vi "scanallvalues_clip.vi"(0 "VISA resource name out":refnum<visa-resource-name>, 1 "nm ch":i32[](array[numeric]), 2 "Voltages values":dbl[](array[numeric]), 3 "Init clip value":i32[](array[numeric]), 4 "base path":path, 5 "error in":errorcluster, 6 "Integration Board IP":string, 7 "L1 Address":i32, 8 "Save test data":bool=TRUE, 9 "Ch burst":i32, 11 "Init att value":i32[](array[numeric])) -> (14 "50%":dbl[][][][](array[numeric]), 15 "L1 min values":i32[](array[numeric])=[180, 378, 779, 1613, 2478, 4286, 5228, 6743], 19 "error out":errorcluster)   [LabVIEW 2009]
uses:
  <instrlib>/Agilent 81150/Agilent 81150.lvlib
  <vilib>/Analysis/NI_AALPro.lvlib
panel:
  out "State":i16
  out "Data out":string="ACK\r\n"
  out "XY Graph":cluster{"Y":dbl[], "Y":dbl[]}[](graph)
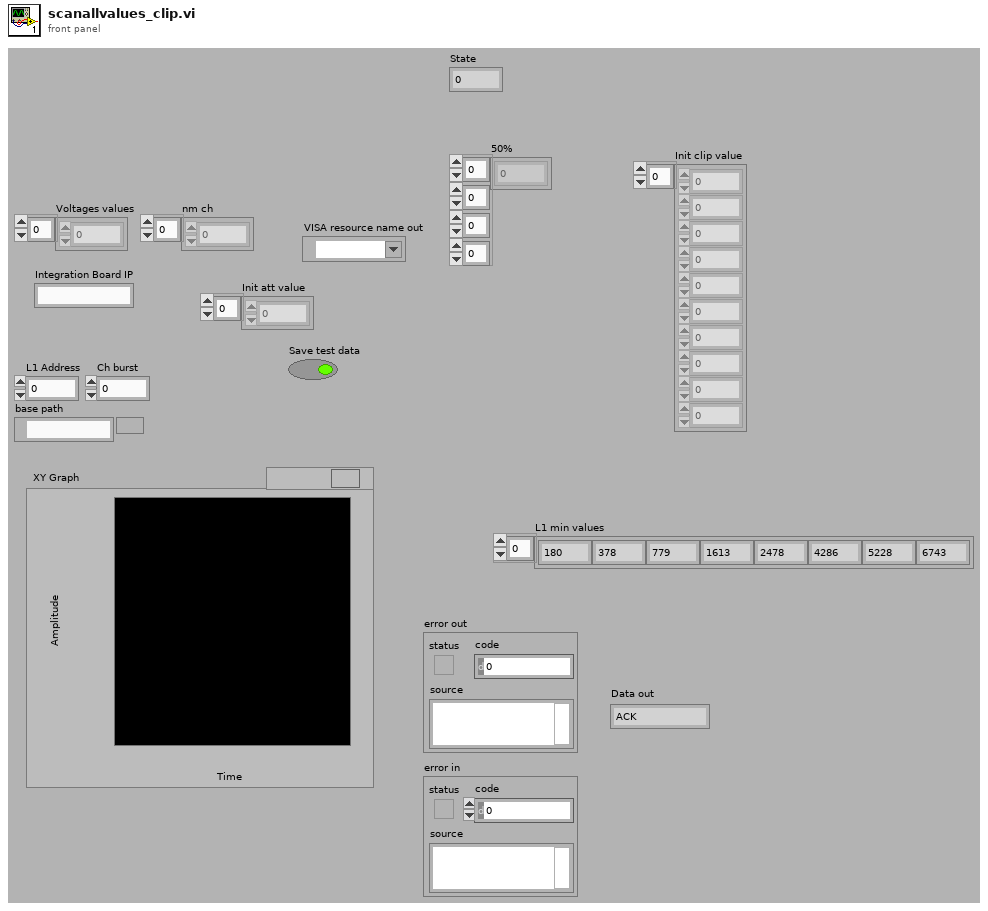
[diagram p1: front panel]
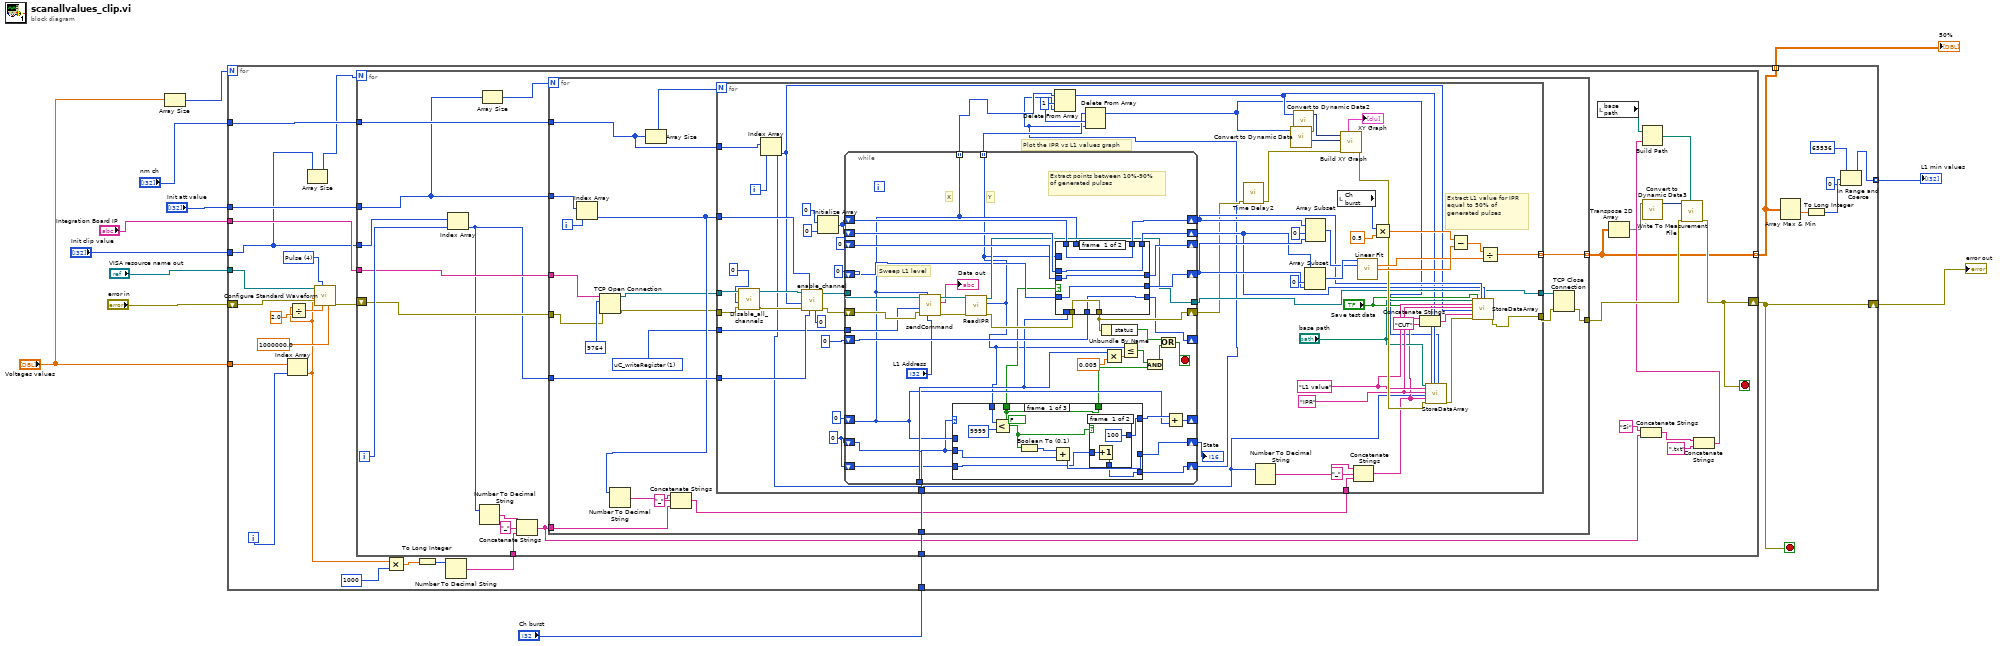
[diagram p0: block diagram]
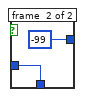
[diagram p2: hidden frame]
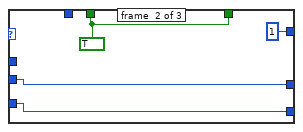
[diagram p3: hidden frame]
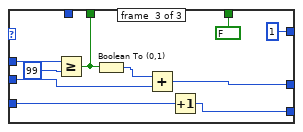
[diagram p4: hidden frame]
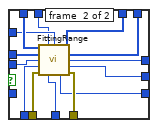
[diagram p5: hidden frame]
diagram:
  n1 = Array Size(array="Voltages values") -> (size(s)=w5:i32)
  n2 = for {
    N: w5 -> [_]
    shift-right: [w26] -> w11
    shift-left: "error in" -> [w25]
    tunnel: [w32] -> w10 mode=indexing
    tunnel: [w28] -> w1 mode=indexing
    tunnel: "Integration Board IP" -> [w27]
    tunnel: "VISA resource name out" -> [w29]
    tunnel: "Voltages values" -> [w19]
    tunnel: "Init clip value" -> [w13]
    tunnel: "Ch burst" -> [w18]
    tunnel: "nm ch" -> [w17]
    tunnel: "Init att value" -> [w15]
    i -> [w34]
    stop <- w26 stop-if-true
    w38 = u16 4 items=["Sine", "Square", "Ramp Up", "Ramp Down", "Pulse", "Noise", "DC"] ("Waveform (0: Sine)")
    n3 = Index Array(array=w19, index=w34) -> (element=w22:dbl)
    n4 = Divide(x=w22, y=2.0) -> (x/y=w36:dbl)
    n5 = Array Size(array=w13) -> (size(s)=w16:i32)
    n6 = call <instrlib>:"Configure Standard Waveform.vi"("Frequency (1000.0 Hz)"=1000000.0, "DC Offset (0.0 Volts)"=w36, "Waveform (0: Sine)"=w38, "error in (no error)"=w25, "Amplitude (1.0 Vpp)"=w22, "VISA resource name"=w29) -> ("error out"=w24:errorcluster)  [unwired: 4 in, 1 out]
    n7 = Multiply(x=w22, y=1000) -> (x*y=w21:dbl)
    n8 = To Long Integer(number=w21) -> (32bit integer=w20:i32)
    n9 = Number To Decimal String(number=w20) -> (decimal integer string=w14:string)  [unwired: 1 in]
    n10 = for {
      N: w16 -> [_]
      tunnel: [w41] -> w28 mode=indexing
      shift-right: [w55] -> w26
      shift-left: w24 -> [w60]
      tunnel: w27 -> [w61]
      tunnel: w13 -> [w43]
      tunnel: w18 -> [w62]
      tunnel: w17 -> [w59]
      tunnel: w15 -> [w42]
      tunnel: w14 -> [w52]
      i -> [w63]
      stop <- w55 stop-if-true
      n11 = Index Array(array=w43, index=w63) -> (element=w54:i32)
      n12 = Number To Decimal String(number=w54) -> (decimal integer string=w51:string)  [unwired: 1 in]
      n13 = Array Size(array=w42) -> (size(s)=w58:i32)
      n14 = Concatenate Strings(w51, "_" ("string"), w52) -> (w44:string)
      n15 = for {
        N: w58 -> [_]
        tunnel: [w84] -> w41 mode=indexing
        tunnel: w62 -> [w83]
        tunnel: [w68] -> w56
        tunnel: w61 -> [w81]
        tunnel: w60 -> [w80]
        tunnel: w59 -> [w76]
        tunnel: w42 -> [w79]
        tunnel: w54 -> [w75]
        tunnel: w44 -> [w73]
        i -> [w78]
        w66 = u16 1 items=["sendCommand"=9, "FPGA_writeRegister"=3, "FPGA_readRegister"=2, "uC_writeRegister"=1, "uC_readRegister"=0] ("Action")
        n16 = Index Array(array=w79, index=w78) -> (element=w74:i32)
        n17 = TCP Open Connection(address=w81, remote port or service name=u16 9764, error in (no error)=w80) -> (connection ID=w64:refnum<k5>, error out=w65:errorcluster)  [unwired: 2 in]
        n18 = Number To Decimal String(number=w74) -> (decimal integer string=w72:string)  [unwired: 1 in]
        n19 = Array Size(array=w76) -> (size(s)=w77:i32)
        n20 = Concatenate Strings(w72, "_" ("string"), w73) -> (w70:string)
        n21 = for {
          N: w77 -> [_]
          tunnel: [w97] -> w84 mode=indexing
          tunnel: w83 -> [w126]
          tunnel: [w123] -> w69
          tunnel: w65 -> [w101]
          tunnel: w64 -> [w100]
          tunnel: w74 -> [w112]
          tunnel: w76 -> [w111]
          tunnel: w75 -> [w109]
          tunnel: w70 -> [w108]
          tunnel: [w104] -> w67
          tunnel: w66 -> [w96]
          i -> [w110]
          w89 = 1 ("length")
          w86 = i16 0
          w132 = "IPR" ("Y Signal Name")
          w133 = "L1 value" ("X Signal Name")
          # "Plot the IPR vs L1 values graph"
          # "Extract L1 value for IPR equal to 50% of generated pulses"
          n22 = call "Disable_all_channels.vi"("error in"=w101, "id_in"=0, "connection ID"=w100) -> ("error out"=w102:errorcluster, "connection ID out"=w99:refnum<k5>)  [unwired: 6 in, 1 out]
          n23 = Index Array(array=w111, index=w110) -> (element=w95:i32)
          n24 = call "enable_channel.vi"("Delay"=0 ("V clip"), "V clip"=w109, "V att"=w112, "error in"=w102, "Channel"=w95, "connection ID"=w99) -> ("error out"=w115:errorcluster, "connection ID out"=w114:refnum<k5>)  [unwired: 3 in, 1 out]
          n25 = Initialize Array(0 ("element"), 0 ("dimension size")) -> (w119:i32[])
          n26 = while {
            tunnel: [w155] -> w88 mode=indexing
            tunnel: [w158] -> w91 mode=indexing
            shift-right: [w182] -> w131
            shift-left: w119 -> [w180]
            shift-right: [w181] -> w130
            shift-left: w119 -> [w179]
            shift-right: [w175] -> w103
            shift-left: w115 -> [w166]
            shift-right: [w177] -> _
            shift-left: 0 ("Array Pointer out") -> [w178]
            tunnel: w114 -> [w167]
            tunnel: [w168] -> w104
            shift-right: [w176] -> w142
            shift-left: 0 ("N_Array Elements") -> [w165]
            shift-right: [w163] -> _
            shift-left: 0 ("State machine") -> [w164]
            tunnel: w126 -> [w162]
            tunnel: w96 -> [w161]
            shift-right: [w160] -> _
            shift-left: 0 ("element") -> [w158]
            shift-right: [w157] -> w94
            shift-left: w86 -> [w154]
            shift-right: [w149] -> w85
            shift-left: w86 -> [w150]
            stop <- w173 stop-if-true
            # "Extract points between 10%-90% of generated pulses"
            # "Sweep L1 level"
            # "Y"
            # "X"
            n27 = call "sendCommand.vi"("Address"="L1 Address", "Data"=w158, "error in"=w166, "Action"=w161, "connection ID"=w167) -> ("error out"=w172:errorcluster, "Data out"=→"Data out":string, "connection ID out"=w171:refnum<k5>)  [unwired: 2 in, 2 out]
            n28 = call "ReadIPR.vi"("error in"=w172, "connection ID"=w171) -> ("error out"=w170:errorcluster, "IPR value"=w155:i32, "connection ID out"=w168:refnum<k5>)  [unwired: 7 in]
            n29 = case shown="0, Default" w154 {
              tunnel: [w194 1 ("x") 1 ("x")] -> w159
              tunnel: w158 -> [_ _ w211]
              tunnel: [w189 w202 w209] -> w157
              tunnel: w154 -> [w190 w202 w208]
              tunnel: [w187 w201 w207] -> w156
              tunnel: w155 -> [w192 _ _]
              tunnel: [w187 w201 FALSE] -> w151
              tunnel: w150 -> [w185 w200 w205]
              tunnel: [w186 w200 w204] -> w149
              frame #0 {
                w187 = FALSE
                n30 = Less?(x=w192, y=9999) -> (x < y?=w188:bool)
                n31 = Boolean To (0,1)(Boolean=w188) -> (0, 1=w191:i16)
                n32 = Add(x=w191, y=w190) -> (x+y=w189:i16)
                n33 = case shown="True" w188 {
                  tunnel: [100 ("x") -99 ("x")] -> w194
                  tunnel: [w196 w198] -> w186
                  tunnel: w185 -> [w195 w198]
                  frame #0 {
                    n34 = Increment(x=w195) -> (x+1=w196:i16)
                  }
                  frame #1 {
                  }
                }
              }
              frame #1 {
                w201 = TRUE
              }
              frame #2 {
                n35 = Greater Or Equal?(x=w211, y=99) -> (x >= y?=w207:bool)
                n36 = Boolean To (0,1)(Boolean=w207) -> (0, 1=w210:i16)
                n37 = Add(x=w210, y=w208) -> (x+y=w209:i16)
                n38 = Increment(x=w205) -> (x+1=w204:i16)
              }
            }
            n39 = case shown="False" w156 {
              tunnel: [w219 w233] -> w182
              tunnel: [w218 w232] -> w181
              tunnel: w180 -> [w219 w231]
              tunnel: w179 -> [w218 w230]
              tunnel: w178 -> [w216 w229]
              tunnel: [w216 w228] -> w177
              tunnel: [w215 w227] -> w176
              tunnel: w162 -> [_ w226]
              tunnel: [w217 w225] -> w175
              tunnel: w170 -> [w217 w224]
              tunnel: w155 -> [_ w223]
              tunnel: w158 -> [_ w222]
              tunnel: w165 -> [w215 _]
              tunnel: w164 -> [w214 w221]
              tunnel: [w214 w220] -> w163
              frame #0 {
              }
              frame #1 {
                n40 = call "FittingRange.vi"("Array in (X)"=w231, "L0 DAC"=w222, "IPR"=w223, "Array in (Y)"=w230, "Array Pointer in"=w229, "Cycles Burst"=w226, "error in"=w224, "State machine"=w221) -> ("Array out (X)"=w233:i32[], "Array out (Y)"=w232:i32[], "Array Pointer out"=w228:i32, "N_Array Elements"=w227:i32, "State machine"=w220:i32, "error out"=w225:errorcluster)  [unwired: 2 in]
              }
            }
            n41 = Unbundle By Name(w175) -> ("status"=w174:bool)
            n42 = Multiply(x=w162, y=0.005) -> (x*y=w183:dbl)
            n43 = Less Or Equal?(x=w155, y=w183) -> (x <= y?=w153:bool)
            n44 = And(x=w153, y=w151) -> (x .and. y?=w152:bool)
            n45 = Or(x=w174, y=w152) -> (x .or. y?=w173:bool)
            n46 = Add(x=w159, y=w158) -> (x+y=w160:i32)
          }
          "State" <- w94
          n47 = Delete From Array(array=w91, length=w89, index=w85) -> (array with subset deleted=w90:i32[])  [unwired: 1 out]
          n48 = Delete From Array(array=w88, length=w89, index=w85) -> (array with subset deleted=w87:i32[])  [unwired: 1 out]
          n49 = call "Time Delay2"("error in (no error)"=w103) -> ("error out"=w122:errorcluster)  [unwired: 10 in]
          n50 = Number To Decimal String(number=w95) -> (decimal integer string=w105:string)  [unwired: 1 in]
          n51 = call "Convert to Dynamic Data"("Array"=w87) -> ("Dynamic Data Type"=w146:dynamicdata)  [unwired: 3 in]
          n52 = call "Convert to Dynamic Data2"("Array"=w90) -> ("Dynamic Data Type"=w145:dynamicdata)  [unwired: 3 in]
          n53 = Array Subset(array=w130, index=0, length=w142) -> (w141:i32[])
          n54 = Array Subset(array=w131, index=0, length=w142) -> (w140:i32[])
          n55 = local read "Ch burst"() -> (w125:i32)
          n56 = call "Build XY Graph"("error in (no error)"=w122, "Y Input"=w146, "X Input"=w145) -> ("error out"=w134:errorcluster, "XY Graph"=→"XY Graph":cluster{"Y":dbl[], "Y":dbl[]}[])  [unwired: 7 in]
          n57 = Concatenate Strings(w105, "_" ("string"), w108) -> (w107:string)
          n58 = call <vilib>:"Linear Fit.vi"("Y"=w141, "X"=w140) -> ("slope"=w135:dbl, "intercept"=w137:dbl)  [unwired: 9 in, 3 out]
          n59 = Multiply(x=w125, y=0.5) -> (x*y=w138:dbl)
          n60 = Concatenate Strings(w107, "CUT" ("string")) -> (w128:string)
          n61 = call "StoreDataArray.vi"("Base path"="base path", "X Signal Name"=w133, "Y Signal Name"=w132, "Channel number"=w95, "Si"=w107, "error in"=w134, "Save test data"="Save test data", "X Array"=w90, "Y Array"=w87) -> ("error out"=w129:errorcluster)  [unwired: 10 in]
          n62 = Subtract(x=w138, y=w137) -> (x-y=w136:dbl)
          n63 = call "StoreDataArray.vi"("Base path"="base path", "X Signal Name"=w133, "Y Signal Name"=w132, "Channel number"=w95, "Si"=w128, "error in"=w129, "Save test data"="Save test data", "X Array"=w131, "Y Array"=w130) -> ("error out"=w123:errorcluster)  [unwired: 10 in]
          n64 = Divide(x=w136, y=w135) -> (x/y=w97:dbl)
        }
        n65 = TCP Close Connection(connection ID=w67, error in (no error)=w69) -> (error out=w68:errorcluster)  [unwired: 1 in, 1 out]
      }
      n66 = local read "base path"() -> (w50:path)
      n67 = Transpose 2D Array(2D array=w41) -> (transposed array=w40:dbl[][])
      n68 = Concatenate Strings("Si" ("string"), w44) -> (w46:string)
      n69 = call "Convert to Dynamic Data3"("2D Array"=w40) -> ("Dynamic Data Type"=w57:dynamicdata)  [unwired: 3 in]
      n70 = Concatenate Strings(w46, ".txt" ("string")) -> (w45:string)
      n71 = Build Path(base path=w50, name or relative path=w45) -> (appended path=w49:path)
      n72 = call "Write To Measurement File"("Signals"=w57, "error in (no error)"=w56, "Filename"=w49) -> ("error out"=w55:errorcluster)  [unwired: 14 in, 2 out]
    }
    n73 = Array Max & Min(array=w28) -> (min value=w35:dbl)  [unwired: 3 out]
    n74 = To Long Integer(number=w35) -> (32bit integer=w33:i32)
    n75 = In Range and Coerce(upper limit=65536, x=w33, lower limit=0) -> (coerced(x)=w32:i32)  [unwired: 1 out]
  }
  "L1 min values" <- w10
  "error out" <- w11
  "50%" <- w1
